vi "Check Syringe Heater Running.vi"(8 "error in (no error)":errorcluster, 11 "cRIO-CO2 in":refnum<class "cRIO-CO2.lvclass">) -> (0 "error out":errorcluster, 1 "Running?":bool, 3 "cRIO-CO2 out":refnum<class "cRIO-CO2.lvclass">)   [LabVIEW 2015, in "cRIO-Carbondioxide.lvlib" / "cRIO-CO2.lvlib" / "cRIO-CO2.lvclass"]
uses:
  cRIO-CO2.lvclass
  <vilib>/ActorFramework/Message Enqueuer/Message Priority.ctl
  cRIO-CO2.lvclass/cRIO-CO2.ctl
  CO2 Actor Messages/Ping Msg/Ping Msg.lvclass/Ping Msg.ctl
  <vilib>/ActorFramework/Message Enqueuer/Message Enqueuer.lvclass/Message Enqueuer.ctl
  <vilib>/ActorFramework/Message Enqueuer/Enqueue.vi
  <vilib>/ActorFramework/Message Priority Queue/Priority Enqueue.vi
  CO2 Actor Messages/Ping Msg/Ping Msg.lvclass
  <vilib>/ActorFramework/Actor/Actor.lvclass
  <vilib>/ActorFramework/Message Enqueuer/Message Enqueuer.lvclass
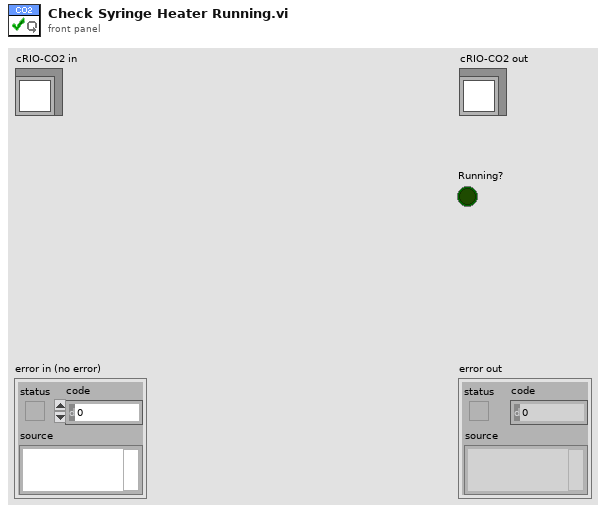
[diagram p1: front panel]
types:
  T1 = typedef "Actor Framework.lvlib/Message Enqueuer.lvclass/Message Priority.ctl" = enum16{"Low", "Normal", "High"}
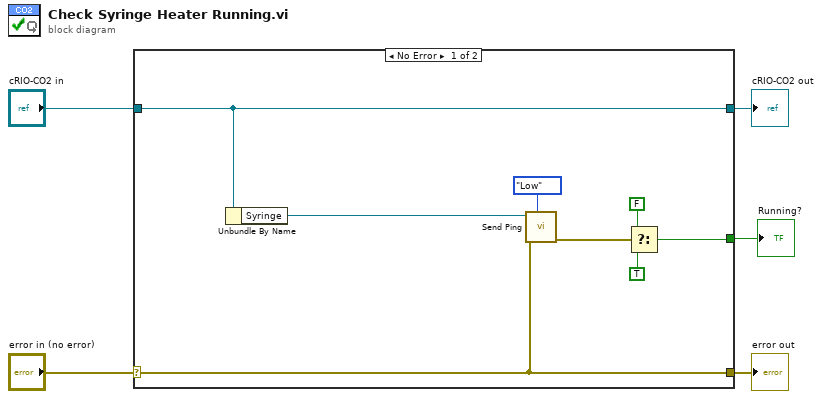
[diagram p0: block diagram]
diagram:
  n1 = case shown="No Error" "error in (no error)" {
    selector: "error in (no error)" -> [w12 w15]
    tunnel: [w12 w15] -> w4
    tunnel: [w13 w14] -> w2
    tunnel: "cRIO-CO2 in" -> [w13 w14]
    tunnel: [w7 _] -> w1
    frame No Error {
      n2 = Unbundle By Name(w13) -> ("Syringe"=w6:refnum<class "Message Enqueuer.lvclass">)
      n3 = call "Send Ping.vi"("Message Priority (Normal)"=Message_Priority."Low", "error in (no error)"=w12, "Message Enqueuer"=w6) -> ("error out"=w10:errorcluster)  [unwired: 5 in, 3 out]
      n4 = Select(t=FALSE, s=w10, f=TRUE) -> (s? t:f=w7:bool)
    }
    frame Error {
    }
  }
  "error out" <- w4
  "cRIO-CO2 out" <- w2
  "Running?" <- w1
